vi "Write Token dur (s).vi"(8 "error in (no error)":errorcluster, 10 "Token dur (s)":dbl, 11 "Noise in":refnum<class "Noise.lvclass">) -> (0 "error out":errorcluster, 3 "Noise out":refnum<class "Noise.lvclass">)   [LabVIEW 2020, in "Noise.lvclass"]
uses:
  Noise.lvclass
  Noise.lvclass/Noise.ctl
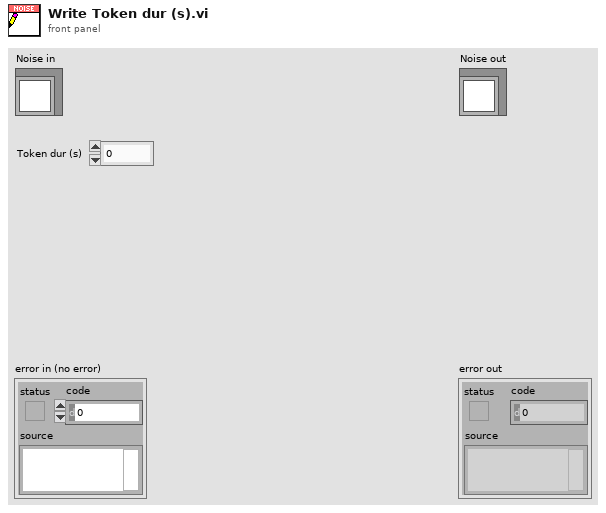
[diagram p1: front panel]
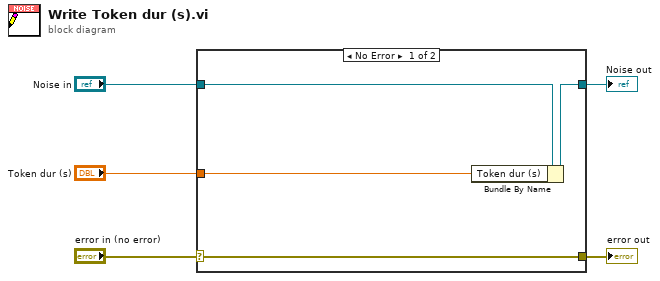
[diagram p0: block diagram]
diagram:
  n1 = case shown="No Error" "error in (no error)" {
    selector: "error in (no error)" -> [w9 w10]
    tunnel: [w9 w10] -> w4
    tunnel: [w7 w11] -> w2
    tunnel: "Noise in" -> [w8 w11]
    tunnel: "Token dur (s)" -> [w6 _]
    frame No Error {
      n2 = Bundle By Name(cluster=w8, "Token dur (s)"=w6) -> (w7:refnum<class "Noise.lvclass">)
    }
    frame Error {
    }
  }
  "error out" <- w4
  "Noise out" <- w2
